vi "io.vi"() -> ()   [LabVIEW 2017]
uses:
  <vilib>/MediaMongrels Ltd/WebSockets/WebSockets/WebSocket Client/WebSocket Client.lvclass
panel:
  out "GetIODO_level":i32
  out "GetIODI_level":i32
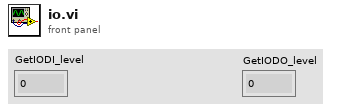
[diagram p1: front panel]
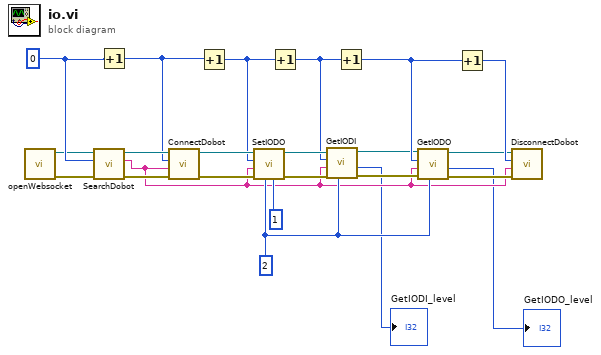
[diagram p0: block diagram]
diagram:
  w18 = 0 ("id")
  w10 = 2 ("port")
  n1 = call <vilib>:"openWebsocket.vi"() -> ("error out"=w3:errorcluster, "WebSocket Client out"=w4:refnum<class "WebSocket Client.lvclass">)  [unwired: 10 in]
  n2 = call <vilib>:"SearchDobot.vi"("error in (no error)"=w3, "id"=w18, "WebSocket in"=w4) -> ("error out"=w20:errorcluster, "portName"=w7:string, "WebSocket out"=w23:refnum<class "WebSocket Client.lvclass">)  [unwired: 6 in]
  n3 = Increment(x=w18) -> (x+1=w17:i32)
  n4 = call <vilib>:"ConnectDobot.vi"("error in (no error)"=w20, "portName"=w7, "id"=w17, "WebSocket in"=w23) -> ("error out"=w19:errorcluster, "WebSocket out"=w22:refnum<class "WebSocket Client.lvclass">)  [unwired: 5 in, 1 out]
  n5 = Increment(x=w17) -> (x+1=w16:i32)
  n6 = call <vilib>:"SetIODO.vi"("level"=1, "port"=w10, "error in (no error)"=w19, "portName"=w7, "id"=w16, "WebSocket in"=w22) -> ("error out"=w12:errorcluster, "WebSocket out"=w13:refnum<class "WebSocket Client.lvclass">)  [unwired: 3 in, 1 out]
  n7 = Increment(x=w16) -> (x+1=w8:i32)
  n8 = call <vilib>:"GetIODI.vi"("port"=w10, "error in (no error)"=w12, "portName"=w7, "id"=w8, "WebSocket in"=w13) -> ("error out"=w11:errorcluster, "level"=→"GetIODI_level":i32, "WebSocket out"=w5:refnum<class "WebSocket Client.lvclass">)  [unwired: 3 in, 1 out]
  n9 = Increment(x=w8) -> (x+1=w9:i32)
  n10 = call <vilib>:"GetIODO.vi"("port"=w10, "error in (no error)"=w11, "portName"=w7, "id"=w9, "WebSocket in"=w5) -> ("error out"=w21:errorcluster, "level"=→"GetIODO_level":i32, "WebSocket out"=w6:refnum<class "WebSocket Client.lvclass">)  [unwired: 3 in, 1 out]
  n11 = Increment(x=w9) -> (x+1=w15:i32)
  n12 = call <vilib>:"DisconnectDobot.vi"("error in (no error)"=w21, "portName"=w7, "id"=w15, "WebSocket in"=w6) -> ()  [unwired: 5 in, 3 out]
